vi "Handle EVENT.vi"(8 "error in (no error)":errorcluster, 9 "Message Loop Data (in)":T1, 10 "Cluster":T16 {"Message Codes" items=["HELLO"=1, "WELCOME"=2, "ABORT"=3, "GOODBYE"=6, "ERROR"=8, "PUBLISH"=16, "PUBLISHED"=17, "SUBSCRIBE"=32, "SUBSCRIBED"=33, "UNSUBSCRIBE"=34, "UNSUBSCRIBED"=35, "EVENT"=36, "CALL"=48, "RESULT"=59, "REGISTER"=64, "REGISTERED"=65, "UNREGISTER"=66, "UNREGISTERED"=67, "INVOCATION"=68, "YIELD"=70]}, 11 "reference":refnum<class "WAMP Client.lvclass">) -> (0 "error out":errorcluster, 1 "Message Loop Data (out)":T1, 3 "reference out":refnum<class "WAMP Client.lvclass">)   [LabVIEW 2020, in "wamplv.lvlib" / "WAMP Client.lvclass"]
uses:
  WAMP Client.lvclass
  TypeDef/WAMP Received Message.ctl
  TypeDef/WAMP Message Codes.ctl
  TypeDef/Message Loop Shift Reg Data.ctl
  TypeDef/REGISTER Request Data.ctl
  API/TypeDefs/INVOCATION payload.ctl
  TypeDef/Success or error.ctl
  API/TypeDefs/Combined error.ctl
  API/TypeDefs/WAMP error.ctl
  TypeDef/Publish Requests Map.ctl
  TypeDef/PUBLISH Request Data.ctl
  TypeDef/PUBLISH result.ctl
  TypeDef/Endpoint Data.ctl
  TypeDef/CALL Request Map.ctl
  TypeDef/CALL Request Data.ctl
  API/TypeDefs/RESULT payload.ctl
  TypeDef/SUBSCRIBE Requests Map.ctl
  TypeDef/SUBSCRIBE Request Data.ctl
  TypeDef/Subscribe Result.ctl
  TypeDef/EVENT payload.ctl
  TypeDef/Subscriptions Map.ctl
  TypeDef/Subscription Details.ctl
  TypeDef/Unsubscribe Requests Map.ctl
  TypeDef/UNSUBSCRIBE Request Data.ctl
  TypeDef/UNSUBSCRIBE Result.ctl
  TypeDef/Unregister requests map.ctl
  TypeDef/Unregister request.ctl
  WAMP Client.lvclass/WAMP Client.ctl
panel:
  out "Details":string
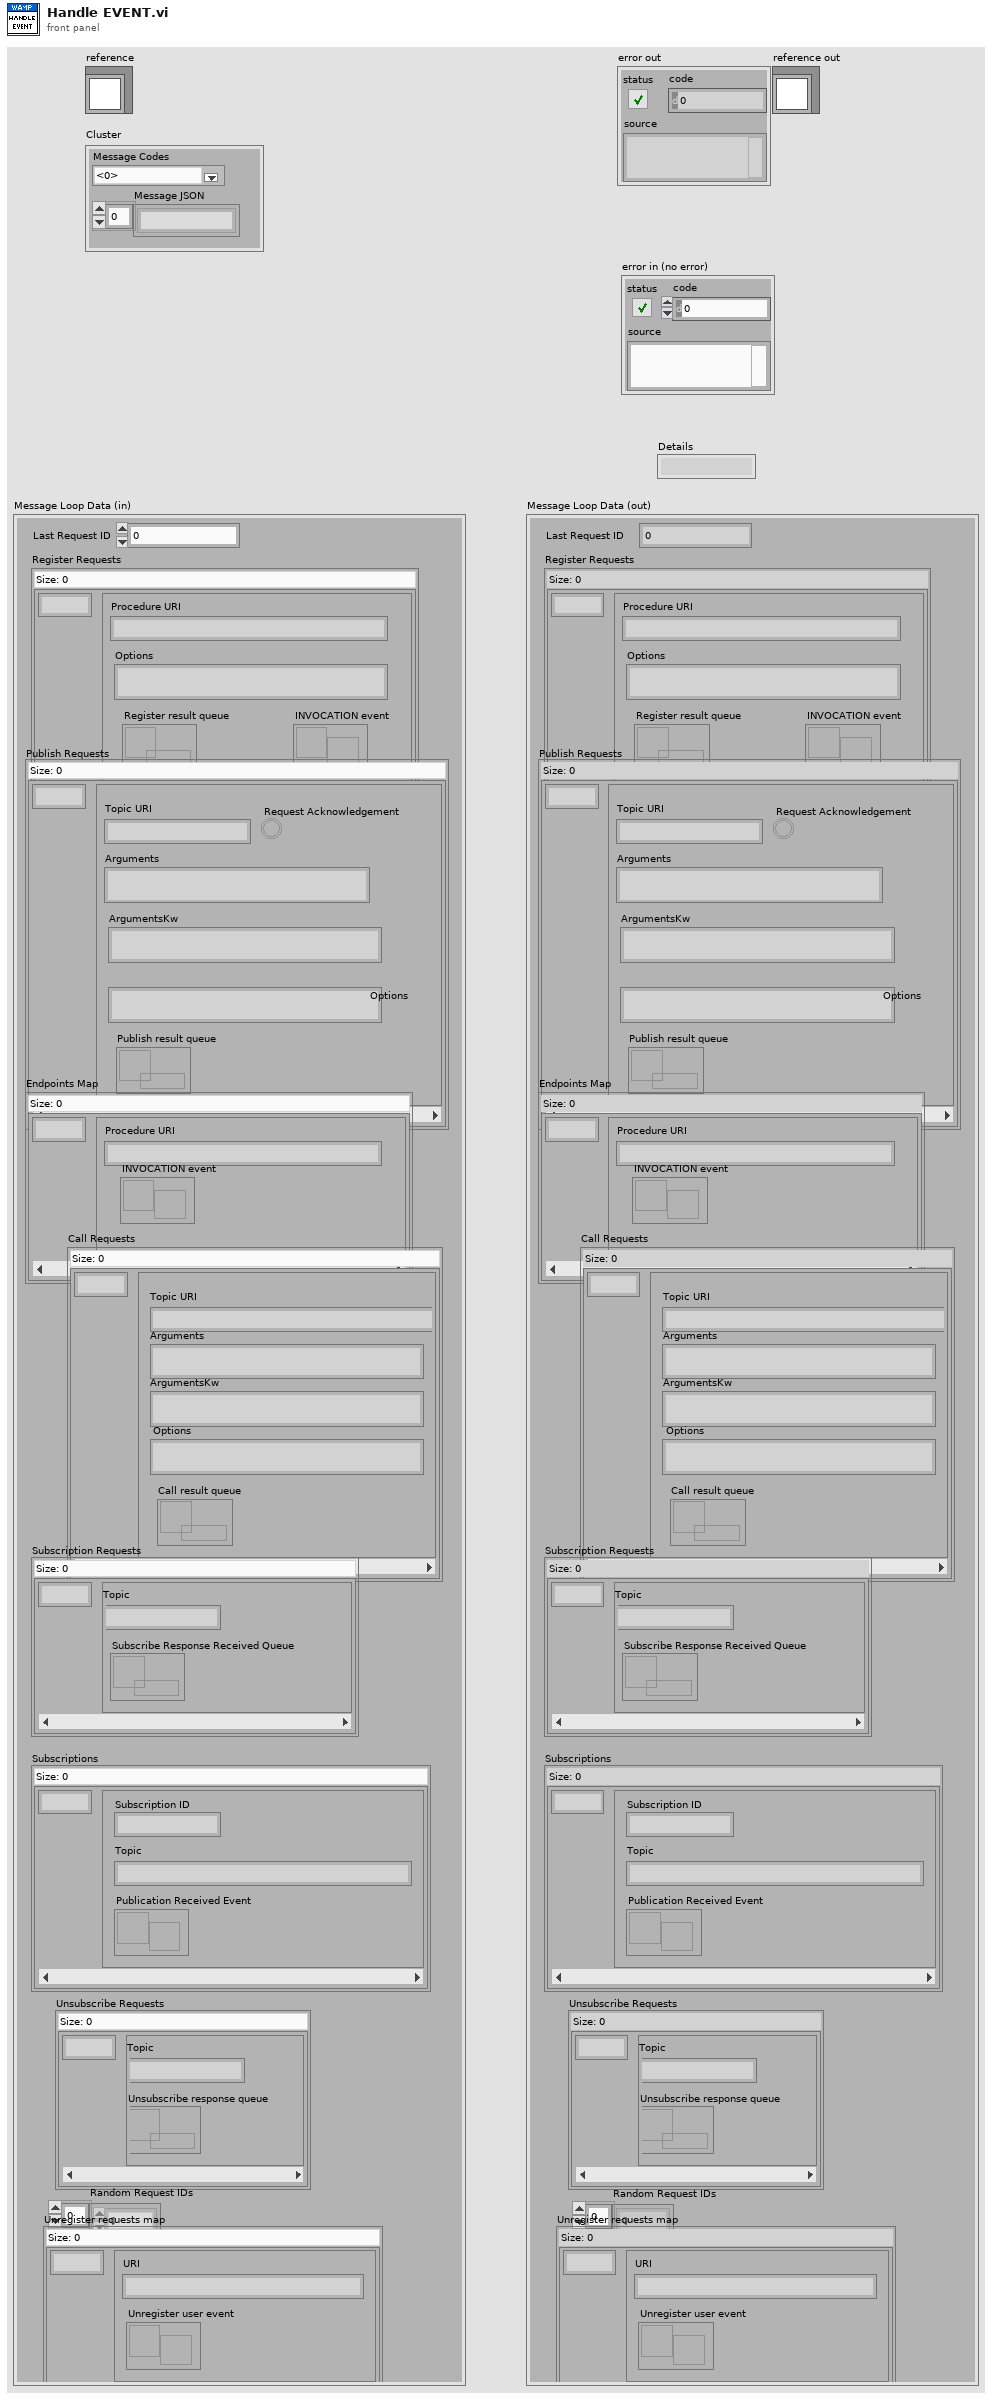
[diagram p1: front panel]
types:
  T1 = typedef "wamplv.lvlib/WAMP Client.lvclass/Message Loop Shift Reg Data.ctl" = cluster{"Last Request ID":u64, "Register Requests":map{u64, T2}, "Publish Requests":T3, "Endpoints Map":map{u64, T5}, "Call Requests":T6, "Subscription Requests":T8, "Subscriptions":T10, "Unsubscribe Requests":T12, "Random Request IDs":u64[], "Unregister requests map":T14}
  T2 = typedef "wamplv.lvlib/WAMP Client.lvclass/REGISTER Request Data.ctl" = cluster{"Procedure URI":string, "Options":string, "INVOCATION event":refnum<user-event>, "Register result queue":refnum<queue>}
  T3 = typedef "wamplv.lvlib/WAMP Client.lvclass/Publish Requests Map.ctl" = map{u64, T4}
  T4 = typedef "wamplv.lvlib/WAMP Client.lvclass/PUBLISH Request Data.ctl" = cluster{"Topic URI":string, "Arguments":string, "ArgumentsKw":string, "Request Acknowledgement":bool, "Options":string, "Publish result queue":refnum<queue>}
  T5 = typedef "wamplv.lvlib/WAMP Client.lvclass/Endpoint Data.ctl" = cluster{"Procedure URI":string, "INVOCATION event":refnum<user-event>}
  T6 = typedef "wamplv.lvlib/WAMP Client.lvclass/CALL Request Map.ctl" = map{u64, T7}
  T7 = typedef "wamplv.lvlib/WAMP Client.lvclass/CALL Request Data.ctl" = cluster{"Topic URI":string, "Arguments":string, "ArgumentsKw":string, "Options":string, "Call result queue":refnum<queue>}
  T8 = typedef "wamplv.lvlib/WAMP Client.lvclass/SUBSCRIBE Requests Map.ctl" = map{u64, T9}
  T9 = typedef "wamplv.lvlib/WAMP Client.lvclass/SUBSCRIBE Request Data.ctl" = cluster{"Topic":string, "Subscribe Response Received Queue":refnum<queue>}
  T10 = typedef "wamplv.lvlib/WAMP Client.lvclass/Subscriptions Map.ctl" = map{u64, T11}
  T11 = typedef "wamplv.lvlib/WAMP Client.lvclass/Subscription Details.ctl" = cluster{"Subscription ID":u64, "Topic":string, "Publication Received Event":refnum<user-event>}
  T12 = typedef "wamplv.lvlib/WAMP Client.lvclass/Unsubscribe Requests Map.ctl" = map{u64, T13}
  T13 = typedef "wamplv.lvlib/WAMP Client.lvclass/UNSUBSCRIBE Request Data.ctl" = cluster{"Topic":string, "Unsubscribe response queue":refnum<queue>}
  T14 = typedef "wamplv.lvlib/WAMP Client.lvclass/Unregister requests map.ctl" = map{u64, T15}
  T15 = typedef "wamplv.lvlib/WAMP Client.lvclass/Unregister request.ctl" = cluster{"URI":string, "Unregister user event":refnum<user-event>}
  T16 = typedef "wamplv.lvlib/WAMP Client.lvclass/WAMP Received Message.ctl" = cluster{"Message JSON":string[], "Message Codes":T17}
  T17 = typedef "wamplv.lvlib/WAMP Client.lvclass/WAMP Message Codes.ctl" = u16
  T18 = typedef "wamplv.lvlib/WAMP Client.lvclass/EVENT payload.ctl" = cluster{"Arguments Payload":string, "ArgumentKw Payload":string, "Topic":string}
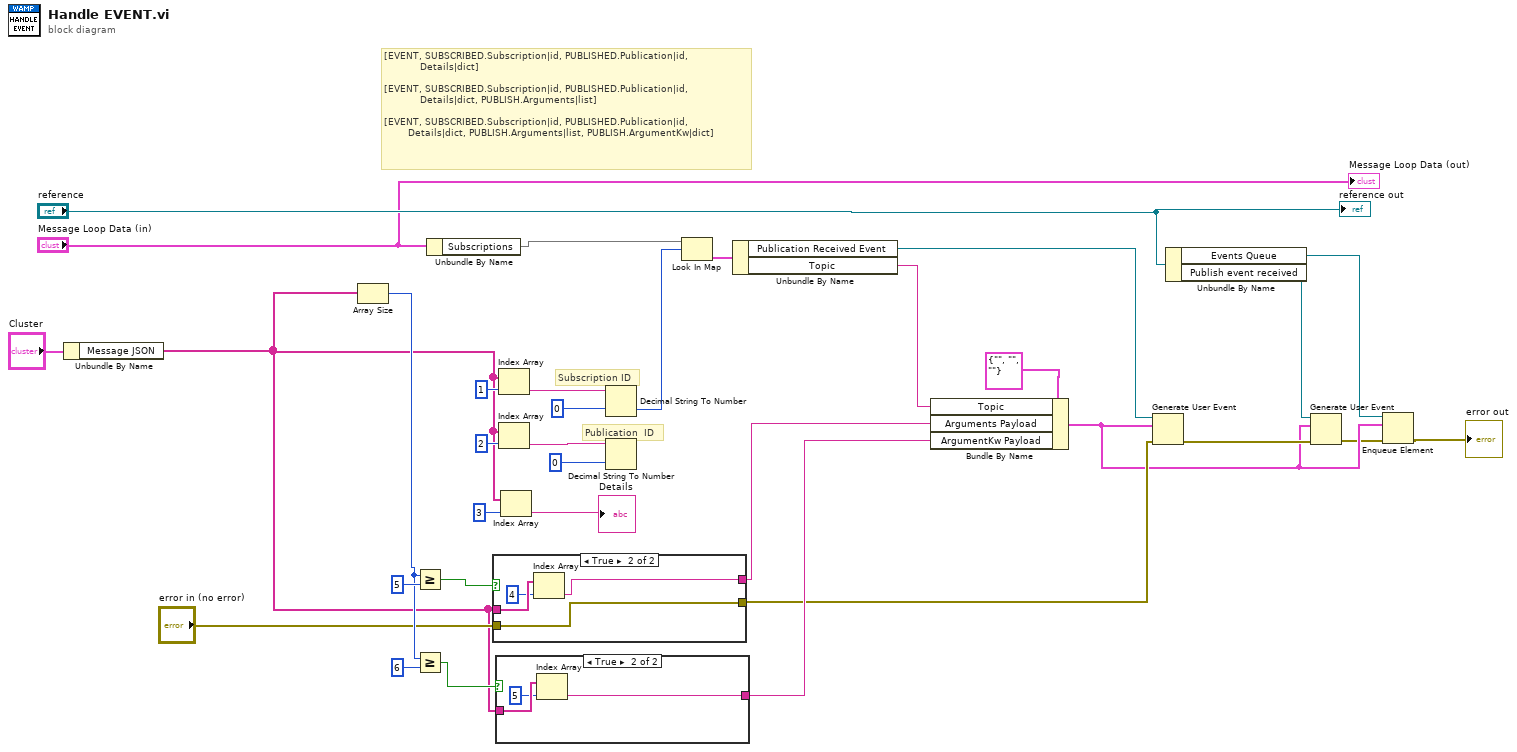
[diagram p0: block diagram]
diagram:
  # "[EVENT, SUBSCRIBED.Subscription|id, PUBLISHED.Publication|id,\n            Details|dict]\n\n[EVENT, SUBSCRIBED.Subscription|id, PUBLISHED.Publication|id,\n            Details|dict, PUBLISH.Arguments|list]\n\n[EVENT, SUBSCRIBED.Subscription|id, PUBLISHED.Publication|id,\n        Details|dict, PUBLISH.Arguments|list, PUBLISH.ArgumentKw|dict]"
  # "Publication  ID"
  # "Subscription ID"
  n1 = Unbundle By Name("Cluster") -> ("Message JSON"=w15:string[])
  n2 = Array Size(array=w15) -> (size(s)=w21:i32)
  n3 = Greater Or Equal?(x=w21, y=5) -> (x >= y?=w24:bool)
  n4 = Greater Or Equal?(x=w21, y=6) -> (x >= y?=w19:bool)
  n5 = Unbundle By Name("Message Loop Data (in)") -> ("Subscriptions"=w2:T10)
  n6 = case shown="True" w24 {
    tunnel: w15 -> [_ w38]
    tunnel: [_ w35] -> w23
    tunnel: "error in (no error)" -> [w34 w36]
    tunnel: [w34 w36] -> w17
    frame False {
    }
    frame True {
      n7 = Index Array(array=w38, index=4) -> (element=w35:string)
    }
  }
  n8 = case shown="True" w19 {
    tunnel: w15 -> [_ w41]
    tunnel: [_ w39] -> w20
    frame False {
    }
    frame True {
      n9 = Index Array(array=w41, index=5) -> (element=w39:string)
    }
  }
  n10 = Index Array(array=w15, index=1) -> (element=w32:string)
  n11 = Index Array(array=w15, index=2) -> (element=w33:string)
  n12 = Index Array(array=w15, index=3) -> (element=→"Details":string)
  n13 = Decimal String To Number(string=w32, default (0L)=u64 0) -> (number=w14:u64)  [unwired: 1 in, 1 out]
  n14 = Decimal String To Number(string=w33, default (0L)=u64 0) -> ()  [unwired: 1 in, 2 out]
  n15 = Look In Map(map=w2, key=w14) -> (value=w13:T11)  [unwired: 1 in, 1 out]
  n16 = Unbundle By Name(w13) -> ("Publication Received Event"=w12:refnum<user-event>, "Topic"=w11:string)
  n17 = Bundle By Name(cluster=T18 {"Arguments Payload"="", "ArgumentKw Payload"="", "Topic"=""} ("Cluster"), "Topic"=w11, "Arguments Payload"=w23, "ArgumentKw Payload"=w20) -> (w5:T18)
  n18 = Generate User Event(user event=w12, event data cluster=w5, error in=w17) -> (error out=w7:errorcluster)  [unwired: 1 in, 1 out]
  n19 = Unbundle By Name("reference") -> ("Events Queue"=w6:refnum<queue>, "Publish event received"=w9:refnum<user-event>)
  n20 = Generate User Event(user event=w9, event data cluster=w5, error in=w7) -> (error out=w4:errorcluster)  [unwired: 1 in, 1 out]
  n21 = Enqueue Element(queue=w6, element=w5, error in (no error)=w4) -> (error out=→"error out":errorcluster)  [unwired: 1 in, 2 out]
  "reference out" <- "reference"
  "Message Loop Data (out)" <- "Message Loop Data (in)"
